vi "CLD 9 Step Sequencer Express Timer Solution2.vi"() -> ()   [LabVIEW 2019]
doc: "CLD 9 Exercise"
uses:
  CLD 9 States2.ctl
  CLD 2 Time Mode.ctl
panel:
  out "Current Step Time":dbl
  out "Elapsed Time (s)":string
  out "Step 3":bool
  out "Step 2":bool
  out "Step 1":bool
  out "Time Has Elapsed":bool
  in  "Auto Reset":bool=TRUE
  in  "Reset Button":bool
  in  "Stop VI":bool
  out "error out":errorcluster
  in  "error in (no error)":errorcluster
  in  "Time Target (s)":dbl
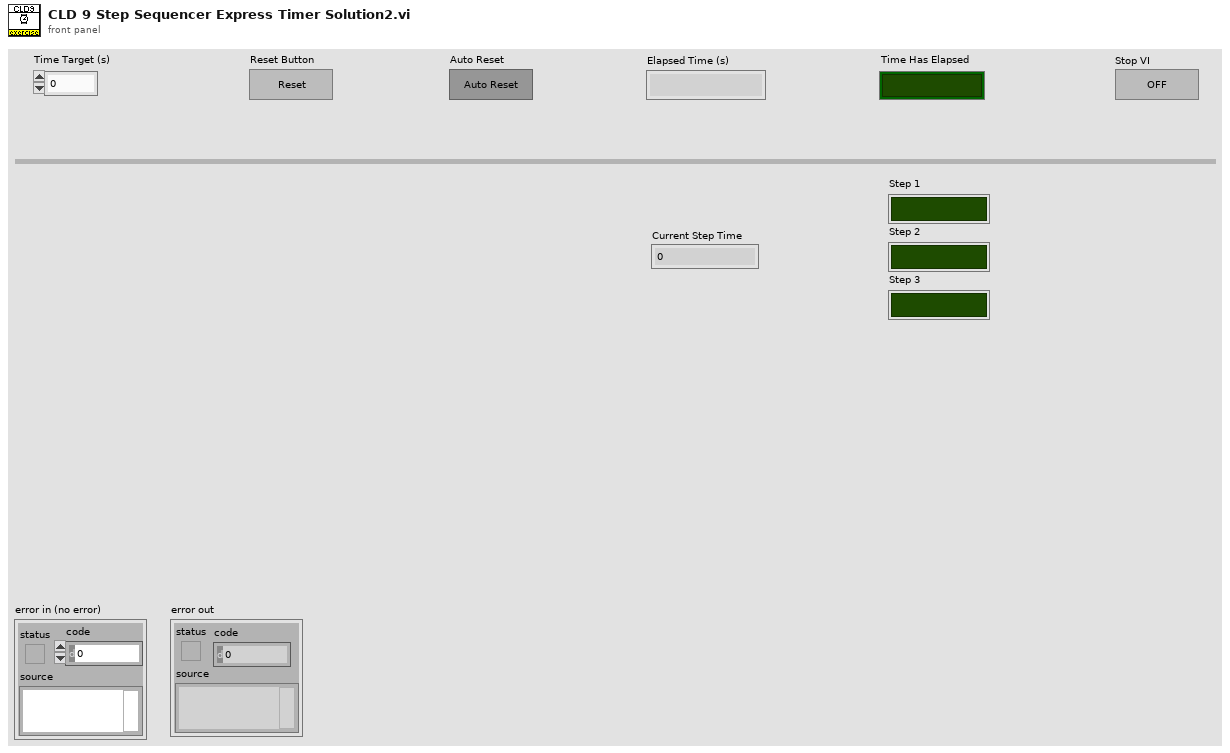
[diagram p1: front panel]
types:
  T1 = typedef "CLD 9 States2.ctl" = enum16{"StartStep", "Step 1", "Step 2", "Step 3"}
  T2 = typedef "CLD 2 Time Mode.ctl" = enum16{"Reset", "Read Status", "Auto Reset and Status", "Update Target"}
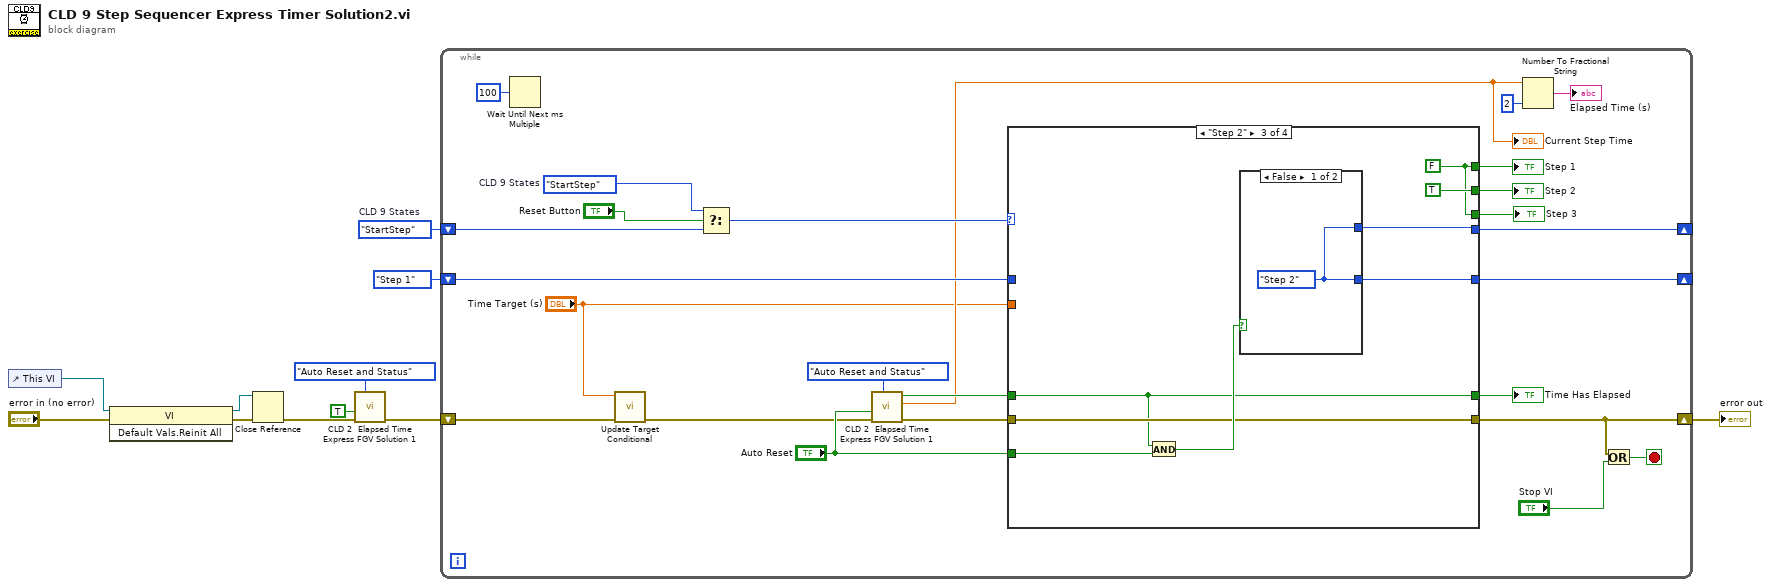
[diagram p0: block diagram]
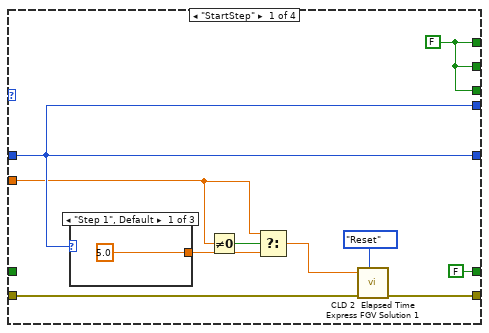
[diagram p2: hidden frame]
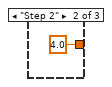
[diagram p3: hidden frame]
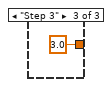
[diagram p4: hidden frame]
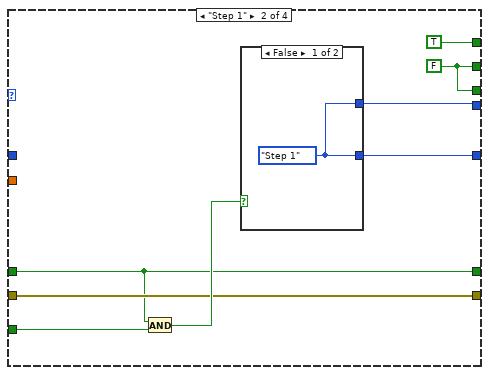
[diagram p5: hidden frame]
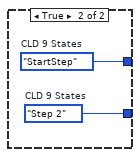
[diagram p6: hidden frame]
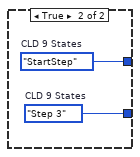
[diagram p7: hidden frame]
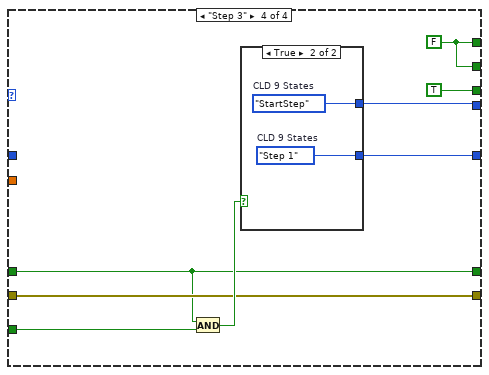
[diagram p8: hidden frame]
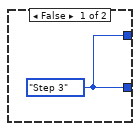
[diagram p9: hidden frame]
diagram:
  w6 = CLD_9_States2."StartStep"  # CLD 9 States
  n1 = control-ref of="This VI"() -> (w9:refnum<vi>)
  n2 = invoke class="VI" method="Default Vals.Reinit All"(reference=w9, error in="error in (no error)") -> (reference out=w8:refnum<vi>, error out=w10:errorcluster)  [unwired: 1 in, 1 out]
  n3 = Close Reference(reference=w8, error in (no error)=w10) -> (error out=w3:errorcluster)
  n4 = call "CLD 2  Elapsed Time Express FGV Solution 1.vi"("Timer  Mode"=CLD_2_Time_Mode."Auto Reset and Status", "error in (no error)"=w3, "Auto Reset (F)"=TRUE) -> ("error out"=w2:errorcluster)  [unwired: 6 in, 2 out]
  n5 = while {
    shift-right: [w35] -> w7
    shift-left: w2 -> [w13]
    shift-right: [w34] -> _
    shift-left: w6 -> [w21]
    shift-right: [w32] -> _
    shift-left: CLD_9_States2."Step 1" ("CLD 9 States") -> [w33]
    stop <- w36 stop-if-true
    w20 = CLD_9_States2."StartStep"  # CLD 9 States
    n6 = Wait Until Next ms Multiple(millisecond multiple=u32 100) -> ()  [unwired: 1 out]
    n7 = call "Update Target Conditional.vi"("error in (no error)"=w13, "Time Target (s)"="Time Target (s)") -> ("error out"=w14:errorcluster)  [unwired: 9 in]
    n8 = Select(t=w20, s="Reset Button", f=w21) -> (s? t:f=w23:T1)
    n9 = call "CLD 2  Elapsed Time Express FGV Solution 1.vi"("Timer  Mode"=CLD_2_Time_Mode."Auto Reset and Status", "error in (no error)"=w14, "Auto Reset (F)"="Auto Reset") -> ("error out"=w18:errorcluster, "Elapsed Time (s)"=w16:dbl, "Time Has Elapsed"=w17:bool)  [unwired: 6 in]
    "Current Step Time" <- w16
    n10 = case shown="\"Step 2\"" w23 {
      tunnel: [w45 w51 w62 w73] -> w35
      tunnel: [w42 w57 w68 w79] -> w34
      tunnel: w33 -> [w42 _ _ _]
      tunnel: [w42 w56 w67 w78] -> w32
      tunnel: [w44 TRUE w63 w75] -> w30
      tunnel: [w44 w54 TRUE w75] -> w29
      tunnel: [w44 w54 w63 TRUE] -> w28
      tunnel: [FALSE ("Time Has Elapsed") w50 w61 w72] -> w26
      tunnel: "Auto Reset" -> [_ w52 w64 w76]
      tunnel: "Time Target (s)" -> [w40 _ _ _]
      tunnel: w18 -> [w37 w51 w62 w73]
      tunnel: w17 -> [_ w50 w61 w72]
      frame "StartStep" {
        w44 = FALSE
        n11 = case shown="\"Step 1\", Default" w42 {
          tunnel: [5.0 ("Time Target (s)") 4.0 ("Time Target (s)") 3.0 ("Time Target (s)")] -> w39
          frame "Step 1", Default {
          }
          frame "Step 2" {
          }
          frame "Step 3" {
          }
        }
        n12 = Not Equal To 0?(x=w40) -> (x != 0?=w41:bool)
        n13 = Select(t=w40, s=w41, f=w39) -> (s? t:f=w38:dbl)
        n14 = call "CLD 2  Elapsed Time Express FGV Solution 1.vi"("Timer  Mode"=CLD_2_Time_Mode."Reset", "error in (no error)"=w37, "Time Target (s)"=w38) -> ("error out"=w45:errorcluster)  [unwired: 6 in, 2 out]
      }
      frame "Step 1" {
        w54 = FALSE
        n15 = And(x=w50, y=w52) -> (x .and. y?=w53:bool)
        n16 = case shown="False" w53 {
          tunnel: [w58 w60] -> w57
          tunnel: [w58 w59] -> w56
          frame False {
            w58 = CLD_9_States2."Step 1" ("CLD 9 States")
          }
          frame True {
            w59 = CLD_9_States2."Step 2"  # CLD 9 States
            w60 = CLD_9_States2."StartStep"  # CLD 9 States
          }
        }
      }
      frame "Step 2" {
        w63 = FALSE
        n17 = And(x=w61, y=w64) -> (x .and. y?=w65:bool)
        n18 = case shown="False" w65 {
          tunnel: [w69 w71] -> w68
          tunnel: [w69 w70] -> w67
          frame False {
            w69 = CLD_9_States2."Step 2" ("CLD 9 States")
          }
          frame True {
            w70 = CLD_9_States2."Step 3"  # CLD 9 States
            w71 = CLD_9_States2."StartStep"  # CLD 9 States
          }
        }
      }
      frame "Step 3" {
        w75 = FALSE
        n19 = And(x=w72, y=w76) -> (x .and. y?=w77:bool)
        n20 = case shown="True" w77 {
          tunnel: [w80 w82] -> w79
          tunnel: [w80 w81] -> w78
          frame False {
            w80 = CLD_9_States2."Step 3" ("CLD 9 States")
          }
          frame True {
            w81 = CLD_9_States2."Step 1"  # CLD 9 States
            w82 = CLD_9_States2."StartStep"  # CLD 9 States
          }
        }
      }
    }
    "Step 1" <- w30
    "Step 2" <- w29
    "Step 3" <- w28
    "Time Has Elapsed" <- w26
    n21 = Number To Fractional String(number=w16, precision (6)=i16 2) -> (F-format string=→"Elapsed Time (s)":string)  [unwired: 2 in]
    n22 = Or(x=w35, y="Stop VI") -> (x .or. y?=w36:bool)
  }
  "error out" <- w7
